vi "extract to time range 3.vi"(8 "error in (no error)":errorcluster, 9 "t0":dbl=-1.0, 10 "t1":dbl=-1.0, 11 "queue in":refnum<queue>) -> (0 "error out":errorcluster, 2 "extracted data":T1[](array[typedef]), 3 "queue out":refnum<queue>)   [LabVIEW 2017]
uses:
  typedefs/reading.ctl
  typedefs/readingType.ctl
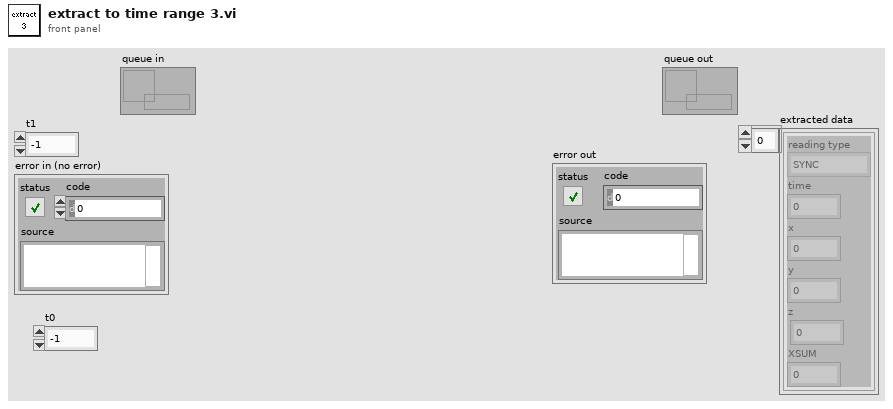
[diagram p1: front panel]
types:
  T1 = typedef "reading.ctl" = cluster{"reading type":T2, "time":fxp<+,48,48>, "x":sgl, "y":sgl, "z":sgl, "XSUM":u8}
  T2 = typedef "readingType.ctl" = enum8{"SYNC", "DETVAL", "COILI", "MAGVEC", "ACCVEC"}
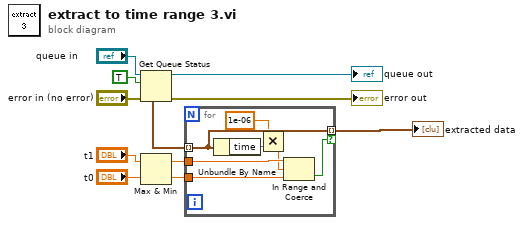
[diagram p0: block diagram]
diagram:
  n1 = Get Queue Status(queue="queue in", return elements? (F)=TRUE, error in (no error)="error in (no error)") -> (queue out=→"queue out":refnum<queue>, error out=→"error out":errorcluster, elements=w10:T1[])  [unwired: 5 out]
  n2 = Max & Min(x="t1", y="t0") -> (max(x,y)=w4:dbl, min(x,y)=w3:dbl)
  n3 = for {
    tunnel: w10 -> [w18] mode=indexing
    tunnel: [w18] -> w7 mode=indexing if=w14
    tunnel: w4 -> [w16]
    tunnel: w3 -> [w15]
    n4 = Unbundle By Name(w18) -> ("time"=w17:fxp<+,48,48>)
    n5 = Multiply(x=1e-06, y=w17) -> (x*y=w13:dbl)
    n6 = In Range and Coerce(upper limit=w16, x=w13, lower limit=w15) -> (In Range?=w14:bool)  [unwired: 1 out]
  }
  "extracted data" <- w7
